vi "setZkAndDofInGroups.vi"(8 "error in (no error)":errorcluster, 9 "DOF in Groups":T1={"M2 Hexapod"=[FALSE, FALSE, FALSE, FALSE, FALSE], "Cam Hexapod "=[FALSE, FALSE, FALSE, FALSE, FALSE], "M1M3 Bending Mode"=[FALSE, FALSE, FALSE, FALSE, FALSE, FALSE, FALSE, FALSE, FALSE, FALSE, FALSE, FALSE, FALSE, FALSE, FALSE, FALSE, FALSE, FALSE, FALSE, FALSE], "M2 Bending Mode"=[FALSE, FALSE, FALSE, FALSE, FALSE, FALSE, FALSE, FALSE, FALSE, FALSE, FALSE, FALSE, FALSE, FALSE, FALSE, FALSE, FALSE, FALSE, FALSE, FALSE]}, 10 "zn3Idx":bool[](array[boolean])=[FALSE, FALSE, FALSE, FALSE, FALSE, FALSE, FALSE, FALSE, FALSE, FALSE, FALSE, FALSE, FALSE, FALSE, FALSE, FALSE, FALSE, FALSE, FALSE], 11 "ZTAAC in":refnum<class "ZTAAC.lvclass">) -> (0 "error out":errorcluster, 3 "ZTAAC out":refnum<class "ZTAAC.lvclass">)   [LabVIEW 2016, in "OfcFunc.lvlib" / "ZTAAC.lvclass"]
doc: "Set the index array of Zk and DOF in groups (M2 hexapod, camera hexapod, M1M3 bending mode, M2 bending mode)."
uses:
  ZTAAC.lvclass
  ZTAAC.lvclass/ZTAAC.ctl
  OptStateEsti/OptStateEsti.lvclass
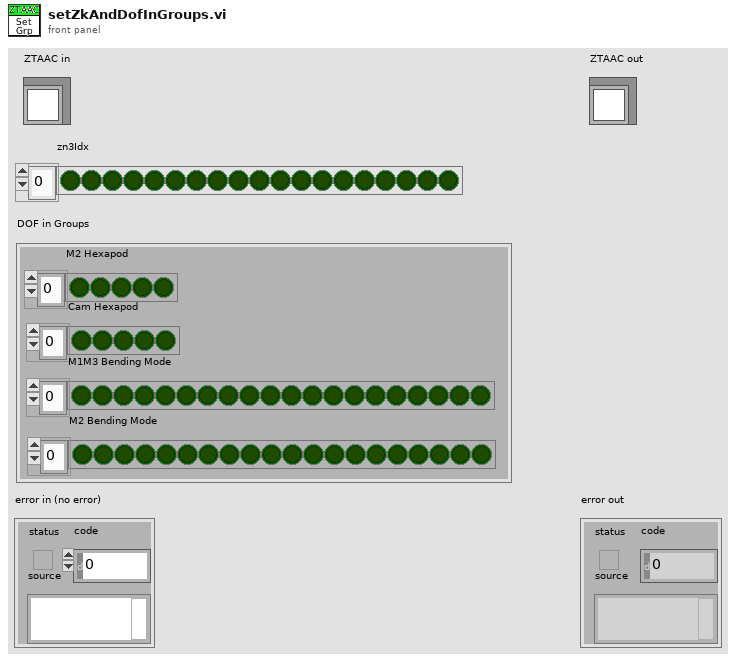
[diagram p1: front panel]
types:
  T1 = cluster{"M2 Hexapod":bool[], "Cam Hexapod ":bool[], "M1M3 Bending Mode":bool[], "M2 Bending Mode":bool[]}
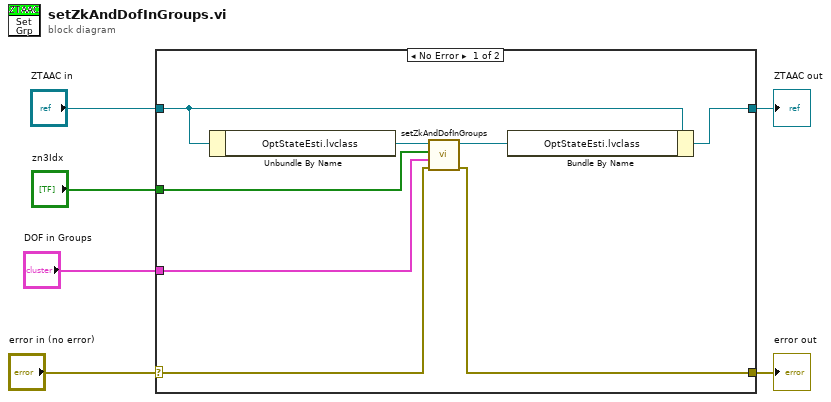
[diagram p0: block diagram]
diagram:
  n1 = case shown="No Error" "error in (no error)" {
    selector: "error in (no error)" -> [w11 w16]
    tunnel: [w10 w16] -> w5
    tunnel: [w7 w15] -> w3
    tunnel: "ZTAAC in" -> [w8 w15]
    tunnel: "zn3Idx" -> [w13 _]
    tunnel: "DOF in Groups" -> [w12 _]
    frame No Error {
      n2 = Unbundle By Name(w8) -> ("OptStateEsti.lvclass"=w14:refnum<class "OptStateEsti.lvclass">)
      n3 = call "setZkAndDofInGroups.vi"("error in (no error)"=w11, "DOF in Groups"=w12, "zn3Idx"=w13, "OptStateEsti in"=w14) -> ("error out"=w10:errorcluster, "OptStateEsti out"=w9:refnum<class "OptStateEsti.lvclass">)  [unwired: 6 in]
      n4 = Bundle By Name(cluster=w8, "OptStateEsti.lvclass"=w9) -> (w7:refnum<class "ZTAAC.lvclass">)
    }
    frame Error {
    }
  }
  "error out" <- w5
  "ZTAAC out" <- w3
